vi "Dot Tracking and SPCM data.vi"(0 "X Parameters":T2={"Number of X Steps"=200, "Max X (V)"=2.0, "Min X (V)"=-2.0}, 1 "X Pos":dbl=192.0, 2 "Scan Interval (minutes)":dbl=7.0, 3 "Y pos":dbl=35.0, 5 "Y Parameters":T1={"Number of Y Steps"=200, "Max Y (V)"=2.0, "Min Y (V)"=-2.0}, 9 "RS232 settings":cluster{"Portnumber":i32, "Baudrate":u16}={"Portnumber"=12, "Baudrate"=5} {"Portnumber" items=["COM1", "COM2", "COM3", "COM4", "COM5", "COM6", "COM7", "COM8", "COM9", "COM10", "COM11", "COM12", "COM13", "COM14", "COM15", "COM16", "COM17", "COM18", "COM19", "COM20", "COM21", "COM22", "COM23", "COM24", "COM25", "COM26", "COM27", "COM28", "COM29", "COM30"]; "Baudrate" items=["9600", "14400", "19200", "38400", "57600", "115200"]}, 11 "Z Position":dbl=52.1, 12 "SPCM File Path":path=path "C:/Users/Ouyang Group/Documents/Calibration pictures/Nanodiamond/8-5-13/X=192 Y=35 1mW 800 sp filter 4 hours.spc", 13 "Collection Time (hours)":dbl=4.0, 14 "Tracking Data File Path":path=path "C:/Users/Ouyang Group/Documents/Calibration pictures/Nanodiamond/8-5-13/X=192 Y=35 1mW 800 sp filter 4 hours position tracking.txt") -> (4 "X Voltage":dbl, 6 "Y Voltage":dbl, 10 "Z Position 2":dbl)   [LabVIEW 2012]
uses:
  <vilib>/DAQmx/write.llb/DAQmx Write (Analog 2D DBL NChan NSamp).vi
  SPCM files/Global FIFO variabls.vi
  <vilib>/Utility/file.llb/Write To Spreadsheet File (DBL).vi
  <vilib>/DAQmx/create/channels.llb/DAQmx Create Channel (AO-Voltage-Basic).vi
  <vilib>/DAQmx/miscellaneous.llb/DAQmx Fill In Error Info.vi
panel:
  out "Intensity":cluster{timestamp[], dbl[]}(graph)
  out "Z Position":cluster{timestamp[], dbl[]}(graph)
  out "Y Position":cluster{timestamp[], dbl[]}(graph)
  out "X Position":cluster{timestamp[], dbl[]}(graph)
  in  "stop":bool
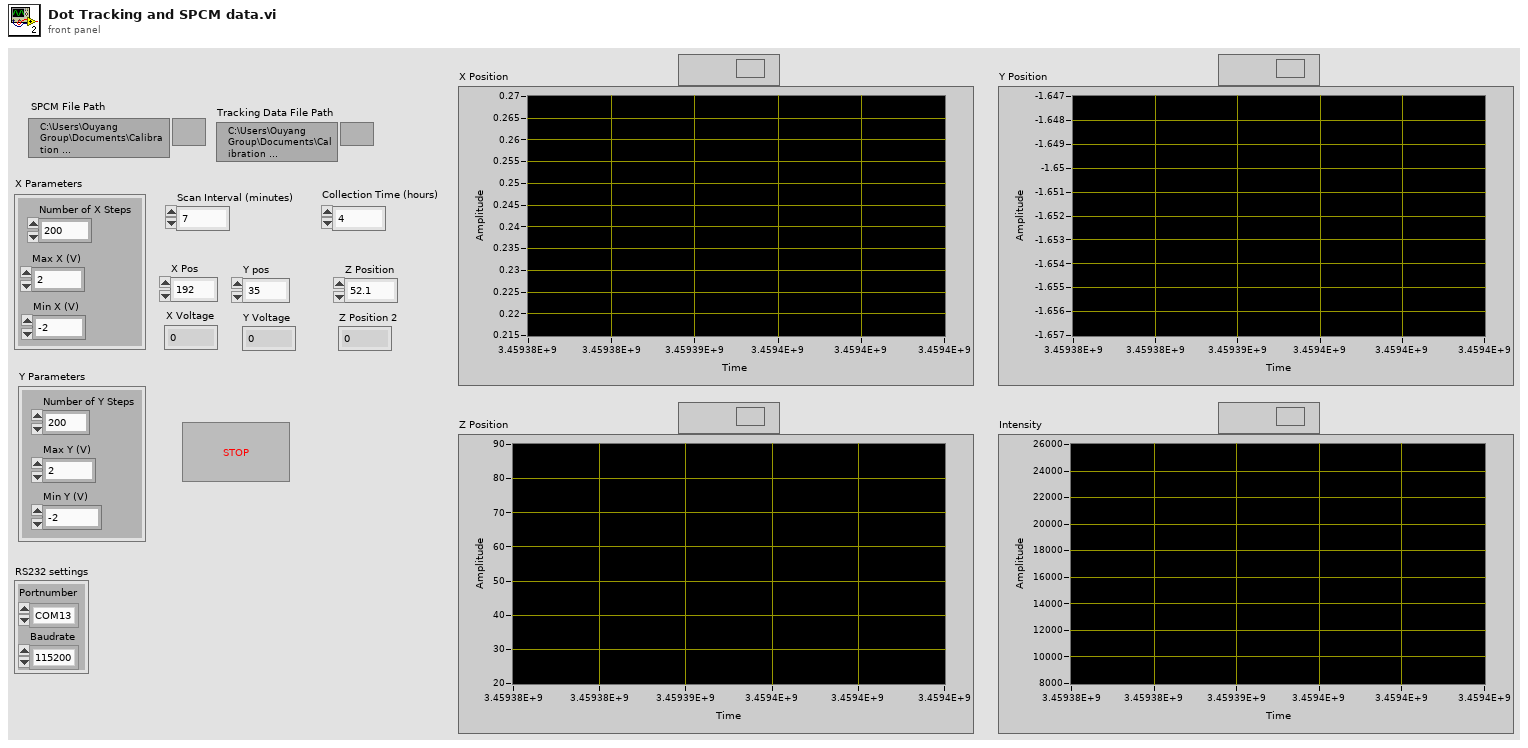
[diagram p1: front panel]
types:
  T1 = cluster{"Number of Y Steps":i32, "Max Y (V)":dbl, "Min Y (V)":dbl}
  T2 = cluster{"Number of X Steps":i32, "Max X (V)":dbl, "Min X (V)":dbl}
  T3 = typedef "error.ctl" = cluster{"Error code":i16, "Message":string}
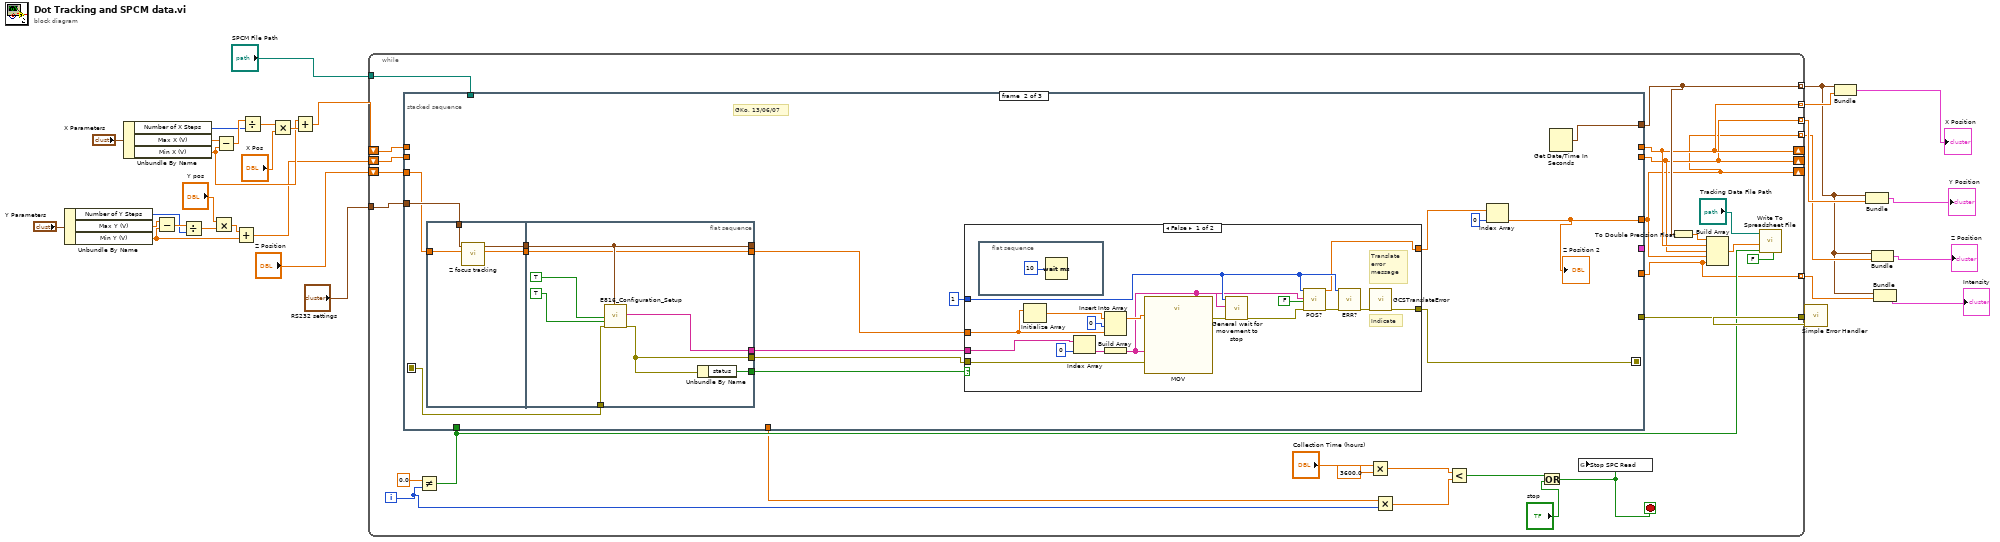
[diagram p0: block diagram]
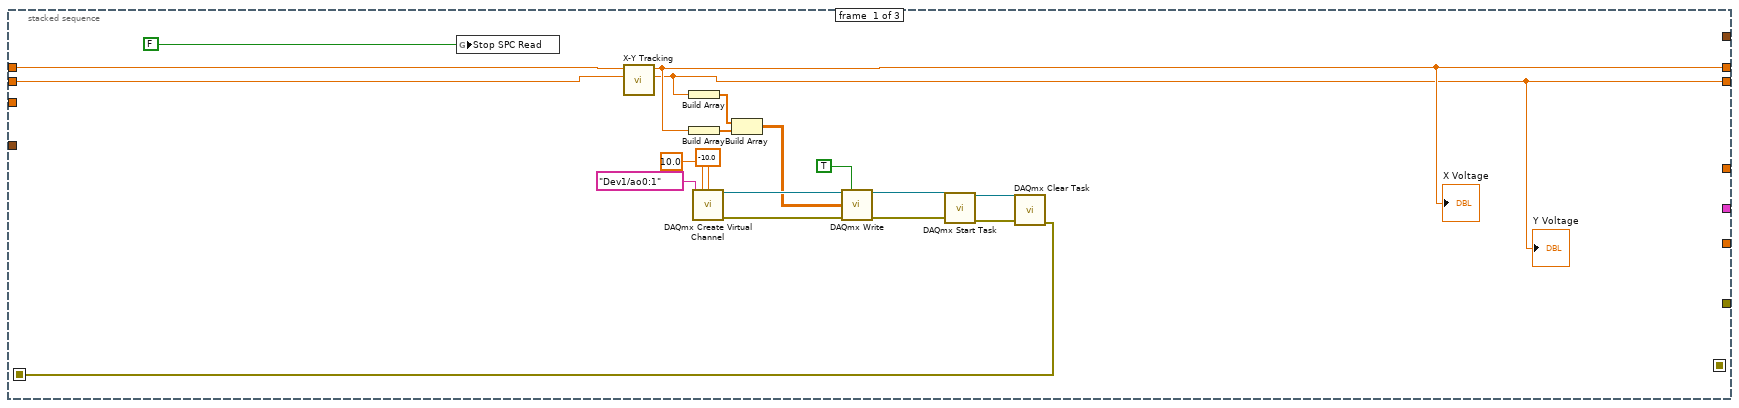
[diagram p2: hidden frame]
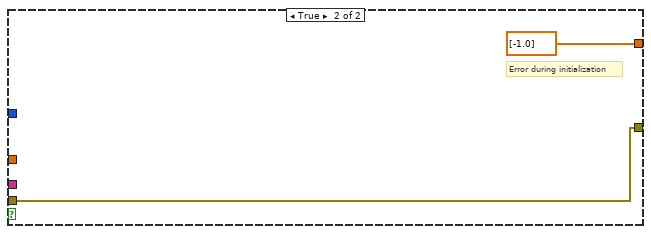
[diagram p3: hidden frame]
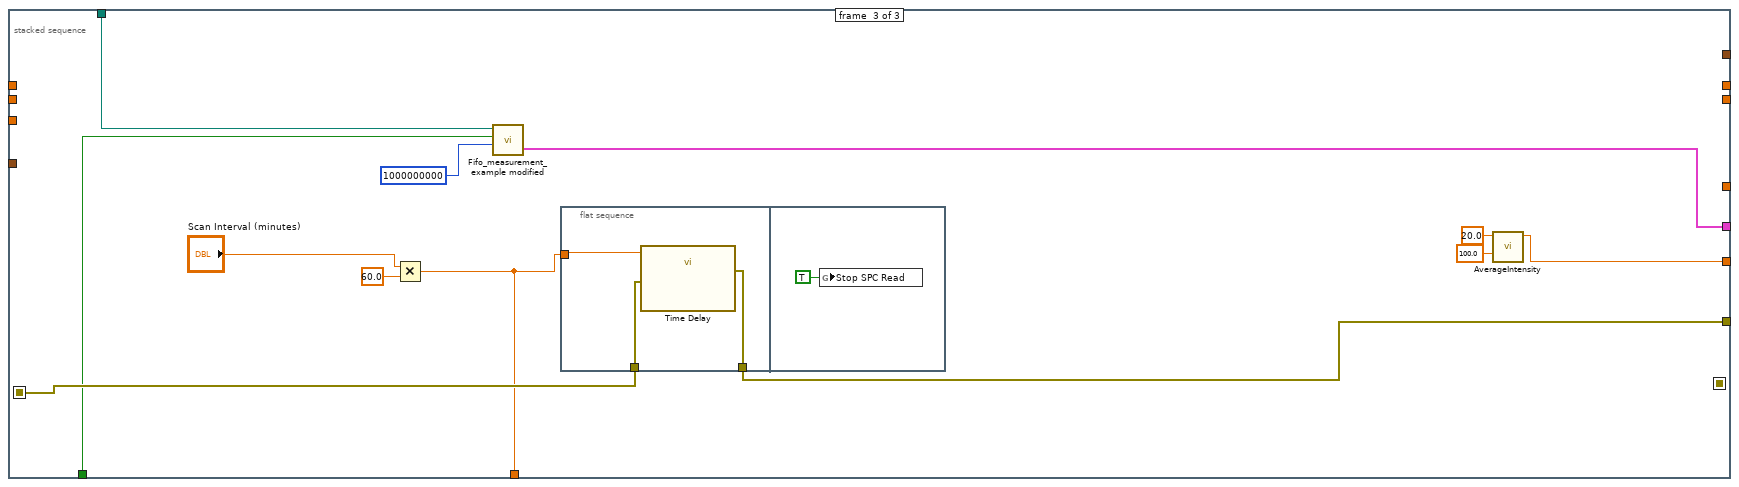
[diagram p4: hidden frame]
diagram:
  n1 = Unbundle By Name("Y Parameters") -> ("Number of Y Steps"=w23:i32, "Max Y (V)"=w22:dbl, "Min Y (V)"=w21:dbl)
  n2 = Unbundle By Name("X Parameters") -> ("Number of X Steps"=w19:i32, "Max X (V)"=w18:dbl, "Min X (V)"=w17:dbl)
  n3 = Subtract(x=w22, y=w21) -> (x-y=w31:dbl)
  n4 = Divide(x=w31, y=w23) -> (x/y=w28:dbl)
  n5 = Multiply(x="Y pos", y=w28) -> (x*y=w27:dbl)
  n6 = Subtract(x=w18, y=w17) -> (x-y=w30:dbl)
  n7 = Add(x=w27, y=w21) -> (x+y=w15:dbl)
  n8 = Divide(x=w30, y=w19) -> (x/y=w25:dbl)
  n9 = Multiply(x=w25, y="X Pos") -> (x*y=w24:dbl)
  n10 = Add(x=w17, y=w24) -> (x+y=w14:dbl)
  n11 = while {
    shift-right: [w44] -> _
    shift-left: w14 -> [w57]
    shift-right: [w43] -> _
    shift-left: w15 -> [w56]
    tunnel: "RS232 settings" -> [w55]
    tunnel: "SPCM File Path" -> [w54]
    shift-right: [w42] -> _
    shift-left: "Z Position" -> [w52]
    tunnel: [w51] -> w10
    tunnel: [w44] -> w6 mode=indexing
    tunnel: [w43] -> w5 mode=indexing
    tunnel: [w42] -> w4 mode=indexing
    tunnel: [w46] -> w2 mode=indexing
    tunnel: [w33] -> w1 mode=indexing
    i -> [w32]
    stop <- w49 stop-if-true
    n12 = Not Equal?(x=0.0, y=w32) -> (x != y?=w38:bool)
    n13 = stacked-sequence {
      seq-local: [_ w90 _] -> [_ _ _]
      seq-local: [w61 _ _] -> [_ w81 w133]
      tunnel: w57 -> [w76 _ _]
      tunnel: w56 -> [w75 _ _]
      tunnel: [w59 _ _] -> w44
      tunnel: [w58 _ _] -> w43
      tunnel: w55 -> [_ w85 _]
      tunnel: w54 -> [_ _ w134]
      tunnel: w38 -> [_ _ w132]
      tunnel: [_ _ w131] -> _
      tunnel: w52 -> [_ w84 _]
      tunnel: [_ w78 _] -> w42
      tunnel: [_ _ w130] -> w51
      tunnel: [_ w77 _] -> w46
      tunnel: [_ _ w126] -> w37
      tunnel: [_ _ w123] -> w33
      frame #0 {
        n14 = global write "Global FIFO variabls.vi" "Stop SPC Read"(FALSE ("Stop SPC Read")) -> ()
        n15 = call "X-Y Tracking.vi"("Y Voltage"=w75, "X Voltage"=w76) -> ("Y centered Voltage"=w58:dbl, "X Centered Voltage"=w59:dbl)  [unwired: 2 in, 6 out]
        "X Voltage" <- w59
        "Y Voltage" <- w58
        n16 = Build Array(w58) -> (w64:dbl[])
        n17 = Build Array(w59) -> (w63:dbl[])
        n18 = call-poly <vilib>:"DAQmx Create Virtual Channel.vi"("maximum value"=10.0, "minimum value"=-10.0, "physical channels"=tag "Dev1/ao0:1") -> ("task out"=w71:refnum<k21>, "error out"=w70:errorcluster)  [unwired: 11 in]
        n19 = Build Array(w64, w63) -> (w62:dbl[][])
        n20 = call-poly <vilib>:"DAQmx Write.vi"("task/channels in"=w71, "auto start"=TRUE, "data"=w62, "error in"=w70) -> ("task out"=w69:refnum<k21>, "error out"=w68:errorcluster)  [unwired: 9 in, 1 out]
        n21 = call <vilib>:"DAQmx Start Task.vi"("task/channels in"=w69, "error in"=w68) -> ("task out"=w67:refnum<k21>, "error out"=w66:errorcluster)  [unwired: 12 in]
        n22 = call <vilib>:"DAQmx Clear Task.vi"("task in"=w67, "error in"=w66) -> ("error out"=w61:errorcluster)  [unwired: 13 in]
      }
      frame #1 {
        # "GKo, 13/06/07"
        n23 = flat-sequence {
          tunnel: [w92] -> w87
          tunnel: [w94] -> w86
          tunnel: w85 -> [w94]
          tunnel: w84 -> [w93]
          tunnel: [w100] -> _
          tunnel: [w95] -> w82
          tunnel: w87 -> [w95]
          tunnel: w86 -> [w100]
          tunnel: [w96] -> w83
          tunnel: w81 -> [w99]
          tunnel: [w98] -> w80
          tunnel: [w97] -> w79
          frame #0 {
            n24 = call "Z focus tracking.vi"("Position"=w93, "RS232 settings"=w94) -> ("center"=w92:dbl)  [unwired: 6 in, 2 out]
          }
          frame #1 {
            n25 = call "E816_Configuration_Setup.vi"("All axes?"=TRUE, "Change servo \nstatus to ON?"=TRUE ("Change servo \nstatus to ON?"), "error in"=w99, "RS232 settings"=w100) -> ("Conn. Axes"=w96:string[], "error out"=w97:errorcluster)  [unwired: 12 in, 2 out]
            n26 = Unbundle By Name(w97) -> ("status"=w98:bool)
          }
        }
        n27 = case shown="False" w80 {
          tunnel: [w118 w122] -> w90
          tunnel: 1 ("System no.") -> [w115 _]
          tunnel: w83 -> [w104 _]
          tunnel: w79 -> [w109 w122]
          tunnel: [w108 dbl[] [-1.0] ("Position")] -> w89
          tunnel: w82 -> [w105 _]
          frame False {
            # "Translate\nerror \nmessage"
            # "Indicate"
            n28 = flat-sequence {
              frame #0 {
                n29 = Wait (ms)(milliseconds to wait=u32 10) -> ()  [unwired: 1 out]
              }
            }
            n30 = Initialize Array(w105) -> (w111:dbl[])  [unwired: 1 in]
            n31 = Index Array(array=w104, index=0) -> (element=w106:string)
            n32 = Insert Into Array(array=w111, index=0, new element=w105) -> (w110:dbl[])
            n33 = Build Array(w106) -> (w103:string[])
            n34 = call "MOV.vi"("Axes to move"=w103, "Position values"=w110, "error in"=w109) -> ("error out"=w113:errorcluster)  [unwired: 16 in]
            n35 = call "General wait for movement to stop.vi"("System no."=w115, "Axes to wait for"=w103, "error in"=w113) -> ("error out"=w114:errorcluster)  [unwired: 15 in, 1 out]
            n36 = call "POS?.vi"("System no."=w115, "Axes to query"=w103, "All axes?"=FALSE, "error in"=w114) -> ("Position"=w108:dbl[], "error out"=w117:errorcluster)  [unwired: 14 in]
            n37 = call "ERR?.vi"("System no."=w115, "error in"=w117) -> ("error out"=w116:errorcluster)  [unwired: 16 in, 1 out]
            n38 = call "GCSTranslateError.vi"("error in"=w116) -> ("error out"=w118:errorcluster)  [unwired: 16 in, 2 out]
          }
          frame True {
            # "Error during initialization"
          }
        }
        n39 = Index Array(array=w89, index=0) -> (element=w78:dbl)
        "Z Position 2" <- w78
        n40 = Get Date/Time In Seconds() -> (seconds since 1Jan1904=w77:timestamp)
      }
      frame #2 {
        n41 = Multiply(x="Scan Interval (minutes)", y=60.0) -> (x*y=w126:dbl)
        n42 = call "Fifo_measurement_example modified.vi"("Required No of photons"=u32 1000000000, "append to file? (new file:F)"=w132, "file path (dialog if empty)"=w134) -> ("SPC error"=w131:T3)  [unwired: 2 in]
        n43 = flat-sequence {
          tunnel: w133 -> [w137]
          tunnel: w126 -> [w136]
          tunnel: [w135] -> w130
          frame #0 {
            n44 = call "Time Delay"("error in (no error)"=w137, "Delay Time (s)"=w136) -> ("error out"=w135:errorcluster)  [unwired: 9 in]
          }
          frame #1 {
            n45 = global write "Global FIFO variabls.vi" "Stop SPC Read"(TRUE ("Stop SPC Read")) -> ()
          }
        }
        n46 = call "AverageIntensity.vi"("rate (Hz)"=100.0, "Time Target (s)"=20.0) -> ("Average intensity (cts/s)"=w123:dbl)  [unwired: 8 in, 1 out]
      }
    }
    n47 = Multiply(x="Collection Time (hours)", y=3600.0) -> (x*y=w35:dbl)
    n48 = Multiply(x=w37, y=w32) -> (x*y=w36:dbl)
    n49 = Less?(x=w35, y=w36) -> (x < y?=w34:bool)
    n50 = Or(x=w34, y="stop") -> (x .or. y?=w49:bool)
    n51 = global write "Global FIFO variabls.vi" "Stop SPC Read"(w49) -> ()
    n52 = To Double Precision Float(number=w46) -> (double precision float=w45:dbl)
    n53 = Build Array(w45, w44, w43, w42, w33) -> (w41:dbl[])
    n54 = call-poly <vilib>:"Write To Spreadsheet File.vi"("transpose? (no:F)"=FALSE, "append to file? (new file:F)"=w38, "1D data"=w41, "file path (dialog if empty)"="Tracking Data File Path") -> ()  [unwired: 4 in, 1 out]
  }
  n55 = call <vilib>:"Simple Error Handler.vi"("error in (no error)"=w10) -> ()  [unwired: 4 in, 5 out]
  n56 = Bundle(w2, w6) -> (→"X Position":cluster{timestamp[], dbl[]})  [unwired: 1 in]
  n57 = Bundle(w2, w5) -> (→"Y Position":cluster{timestamp[], dbl[]})  [unwired: 1 in]
  n58 = Bundle(w2, w4) -> (→"Z Position":cluster{timestamp[], dbl[]})  [unwired: 1 in]
  n59 = Bundle(w2, w1) -> (→"Intensity":cluster{timestamp[], dbl[]})  [unwired: 1 in]
